vi "Project Folder.vi"(8 "error in (no error)":errorcluster, 9 "Request File Name":string, 10 "Revision":i32, 11 "Method":string) -> (0 "error out":errorcluster, 3 "Completed Design path":path)   [LabVIEW 2015]
uses:
  Folders.ctl
  Design Server.lvlib
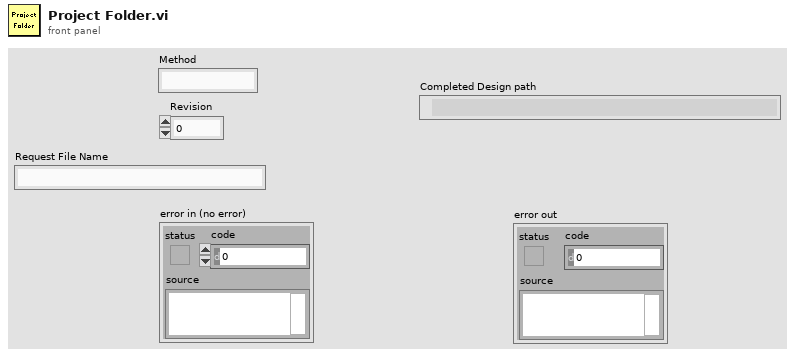
[diagram p1: front panel]
types:
  T1 = typedef "Design Server.lvlib/Folders.ctl" = enum16{"MathcadMethods", "RequestedDesigns", "CompletedDesigns", "MathcadCode", "CollabnetSVN.exe"}
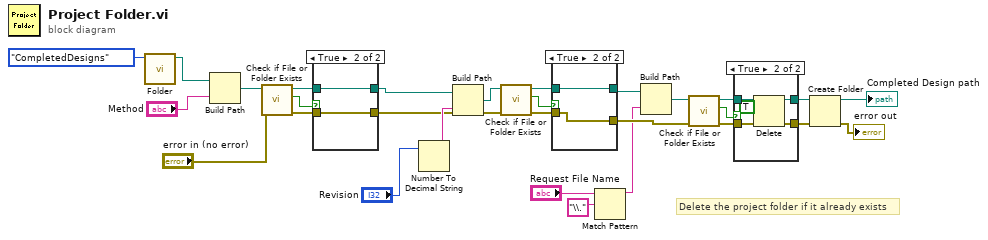
[diagram p0: block diagram]
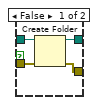
[diagram p3: hidden frame]
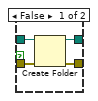
[diagram p4: hidden frame]
diagram:
  # "Delete the project folder if it already exists"
  n1 = call "Folder.vi"("Folders"=Folders."CompletedDesigns") -> ("FolderPath"=w28:path)  [unwired: 8 in, 2 out]
  n2 = Build Path(base path=w28, name or relative path="Method") -> (appended path=w26:path)
  n3 = call <vilib>:"Check if File or Folder Exists.vi"("error in (no error)"="error in (no error)", "path"=w26) -> ("error out"=w24:errorcluster, "file or folder exists?"=w25:bool, "dup path"=w23:path)  [unwired: 7 in]
  n4 = case shown="True" w25 {
    tunnel: w24 -> [w33 w34]
    tunnel: w23 -> [w32 w35]
    tunnel: [w31 w35] -> w22
    tunnel: [w30 w34] -> w17
    frame False {
      n5 = Create Folder(path (use dialog)=w32, error in=w33) -> (created path=w31:path, error out=w30:errorcluster)  [unwired: 1 in, 1 out]
    }
    frame True {
    }
  }
  n6 = Number To Decimal String(number="Revision") -> (decimal integer string=w21:string)  [unwired: 1 in]
  n7 = Build Path(base path=w22, name or relative path=w21) -> (appended path=w18:path)
  n8 = call <vilib>:"Check if File or Folder Exists.vi"("error in (no error)"=w17, "path"=w18) -> ("error out"=w19:errorcluster, "file or folder exists?"=w15:bool, "dup path"=w16:path)  [unwired: 7 in]
  n9 = case shown="True" w15 {
    tunnel: w19 -> [w39 w40]
    tunnel: w16 -> [w38 w41]
    tunnel: [w37 w41] -> w10
    tunnel: [w36 w40] -> w9
    frame False {
      n10 = Create Folder(path (use dialog)=w38, error in=w39) -> (created path=w37:path, error out=w36:errorcluster)  [unwired: 1 in, 1 out]
    }
    frame True {
    }
  }
  n11 = Match Pattern(string="Request File Name", regular expression="\\.") -> (before substring=w5:string)  [unwired: 1 in, 3 out]
  n12 = Build Path(base path=w10, name or relative path=w5) -> (appended path=w12:path)
  n13 = call <vilib>:"Check if File or Folder Exists.vi"("error in (no error)"=w9, "path"=w12) -> ("error out"=w11:errorcluster, "file or folder exists?"=w14:bool, "dup path"=w13:path)  [unwired: 7 in]
  n14 = case shown="True" w14 {
    tunnel: w11 -> [w42 w47]
    tunnel: w13 -> [w43 w48]
    tunnel: [w43 w46] -> w3
    tunnel: [w42 w45] -> w4
    frame False {
    }
    frame True {
      n15 = Delete(path (use dialog)=w48, entire hierarchy (F)=TRUE, error in=w47) -> (deleted path=w46:path, error out=w45:errorcluster)  [unwired: 2 in, 1 out]
    }
  }
  n16 = Create Folder(path (use dialog)=w3, error in=w4) -> (created path=→"Completed Design path":path, error out=→"error out":errorcluster)  [unwired: 1 in, 1 out]
